vi "Load Becker-Hickl FLIM Data.vi"(4 "Data Block Idx":i32, 6 "Image Sizes":T1, 8 "error in (no error)":errorcluster, 9 "# Data Blocks":i16, 10 "Data Block Offset":i32, 11 "File Path":path) -> (0 "error out":errorcluster, 3 "Data":sgl[][][](array[numeric]))   [LabVIEW 2021, in "Becker-Hickl Files.lvlib"]
uses:
  Becker-Hickl Files.lvlib
  Becker-Hickl FLIM Image Sizes.ctl
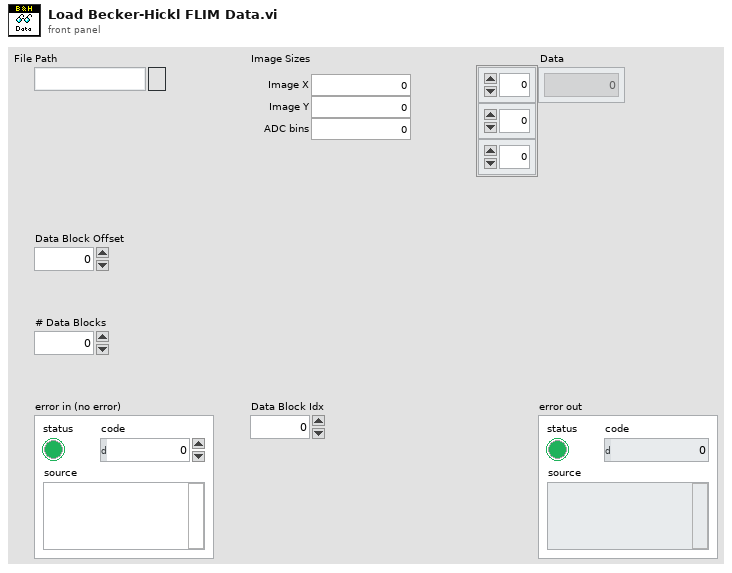
[diagram p1: front panel]
types:
  T1 = typedef "Becker-Hickl Files.lvlib/Becker-Hickl FLIM Image Sizes.ctl" = cluster{"Image X":i32, "Image Y":i32, "ADC bins":i32}
  T2 = typedef "Becker-Hickl Files.lvlib/Becker-Hickl Data Block Type.ctl" = cluster{"Creation Mode":T3, "Block Content":T4, "Data Type":T5}
  T3 = typedef "Becker-Hickl Files.lvlib/Becker-Hickl Data Creation Mode.ctl" = enum16{"NOT_USED", "MEAS_DATA", "FLOW_DATA", "MEAS_DATA_FROM_FILE", "CALC_DATA", "SIM_DATA", "FIFO_DATA", "FIFO_DATA_FROM_FILE"}
  T4 = typedef "Becker-Hickl Files.lvlib/Becker-Hickl Data Block Content.ctl" = enum16{"DECAY_BLOCK", "PAGE_BLOCK", "FCS_BLOCK", "FIDA_BLOCK", "FILDA_BLOCK", "MCS_BLOCK", "IMG_BLOCK"}
  T5 = typedef "Becker-Hickl Files.lvlib/Becker-Hickl Data Type.ctl" = enum16{"DATA_USHORT", "DATA_ULONG", "DATA_DBL"}
  T6 = typedef "Becker-Hickl Files.lvlib/Becker-Hickl Data Block Header.ctl" = cluster{"Block Number":u16, "Data Offset":u32, "Next Block Offset":u32, "Block Type":u16, "Measurement Description Block Number":u16, "Long Block Number":u32, "Block Length":u32}
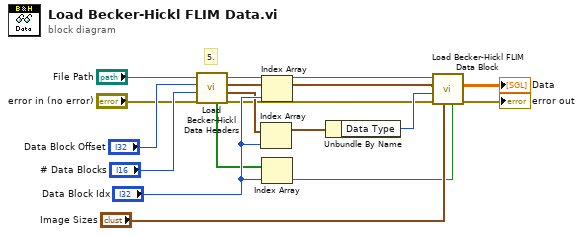
[diagram p0: block diagram]
diagram:
  # "5."
  n1 = call "Load Becker-Hickl Data Headers.vi"("Error In"="error in (no error)", "# Data Blocks"="# Data Blocks", "Data Block Offset"="Data Block Offset", "File Path Control"="File Path") -> ("Error Out"=w5:errorcluster, "Data Block Types"=w15:T2[], "Data Block Headers"=w9:T6[], "File Path"=w8:path, "Compressed"=w12:bool[])  [unwired: 3 in]
  n2 = Index Array(array=w15, index="Data Block Idx") -> (element=w14:T2)
  n3 = Index Array(array=w9, index="Data Block Idx") -> (element=w10:T6)
  n4 = Index Array(array=w12, index="Data Block Idx") -> (element=w13:bool)
  n5 = Unbundle By Name(w14) -> ("Data Type"=w11:T5)
  n6 = call "Load Becker-Hickl FLIM Data Block.vi"("Compressed?"=w13, "Image Sizes"="Image Sizes", "Error In"=w5, "Data Type"=w11, "Data Block Header"=w10, "File Path Control"=w8) -> ("Error Out"=→"error out":errorcluster, "Data"=→"Data":sgl[][][])  [unwired: 3 in, 1 out]
